vi "Copy.vi"(5 "XRef":refnum<vi>, 6 "State In":T1) -> (0 "Reply":string[](array[string]), 2 "State Out":T1)   [LabVIEW 2010, in "CData Flatten XNode.xnode"]
doc: "This ability VI is called by LabVIEW after the user copies an XNode. State In is the same as the original XNode's state. The generated code is copied from the old XNode and will not be regenerated unless you return the GenerateCode reply.\n\nDefault behavior: Produce an exact copy of the original XNode without regenerating the code.\n\nThis ability does not provide UI and OS messages are not handled.\n\nSee also: Initialize"
uses:
  CData Flatten XNode.xnode
  State.ctl
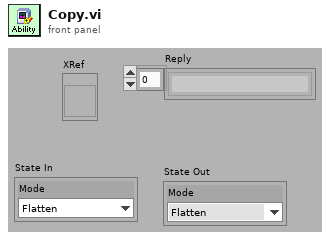
[diagram p1: front panel]
types:
  T1 = typedef "CData Flatten XNode.xnode/State.ctl" = cluster{"Mode":enum16{"Flatten", "Unflatten"}}
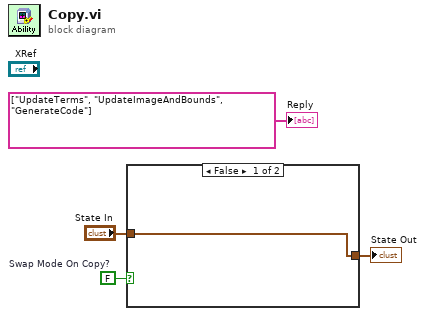
[diagram p0: block diagram]
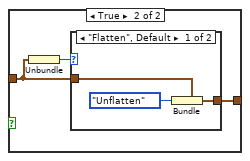
[diagram p2: hidden frame]
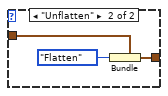
[diagram p3: hidden frame]
diagram:
  w2 = FALSE  # Swap Mode On Copy?
  n1 = case shown="False" w2 {
    tunnel: [w5 w7] -> w4
    tunnel: "State In" -> [w5 w6]
    frame False {
    }
    frame True {
      n2 = Unbundle(w6) -> ("Mode"=w8:enum16{"Flatten", "Unflatten"})
      n3 = case shown="\"Flatten\", Default" w8 {
        tunnel: [w9 w13] -> w7
        tunnel: w6 -> [w11 w14]
        frame "Flatten", Default {
          n4 = Bundle(cluster=w11, "Mode"=enum16{"Flatten", "Unflatten"}."Unflatten") -> (w9:T1)
        }
        frame "Unflatten" {
          n5 = Bundle(cluster=w14, "Mode"=enum16{"Flatten", "Unflatten"}."Flatten") -> (w13:T1)
        }
      }
    }
  }
  "State Out" <- w4
  "Reply" <- string[] ["UpdateTerms", "UpdateImageAndBounds", "GenerateCode"] ("Reply")
